vi "Read Drop_out.vi"(8 "error in (no error)":errorcluster, 11 "EVI 79 in":refnum<class "EVI 79.lvclass">) -> (0 "error out":errorcluster, 2 "Drop_out":T1={"V"=24.0, "I"=0.5, "V_reduced"=4.0, "V_perturb"=0.01, "Plunger_Threshold"=0.01, "V_MIN"=0.01}, 3 "EVI 79 out":refnum<class "EVI 79.lvclass">)   [LabVIEW 2025, in "EVI 79.lvclass"]
uses:
  EVI 79.lvclass
  EVI 79.lvclass/EVI 79.ctl
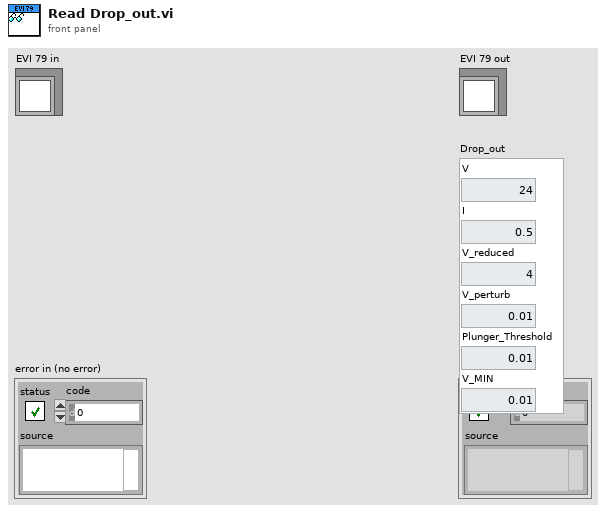
[diagram p1: front panel]
types:
  T1 = cluster{"V":dbl, "I":dbl, "V_reduced":dbl, "V_perturb":dbl, "Plunger_Threshold":dbl, "V_MIN":dbl}
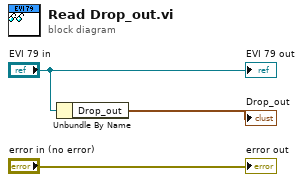
[diagram p0: block diagram]
diagram:
  n1 = Unbundle By Name("EVI 79 in") -> ("Drop_out"=→"Drop_out":T1)
  "error out" <- "error in (no error)"
  "EVI 79 out" <- "EVI 79 in"
